vi "Write SAL_Events.vi"(8 "error in (no error)":errorcluster, 10 "SAL_Events.lvclass":refnum<class "SAL_Events.lvclass">, 11 "SAL_Listener in":refnum<class "SAL_Listener.lvclass">) -> (0 "error out":errorcluster, 3 "SAL_Listener out":refnum<class "SAL_Listener.lvclass">)   [LabVIEW 2016, in "SAL_Listener.lvclass"]
uses:
  SAL_Listener.lvclass
  SALEvents/SAL_Events.lvclass
  SAL_Listener.lvclass/SAL_Listener.ctl
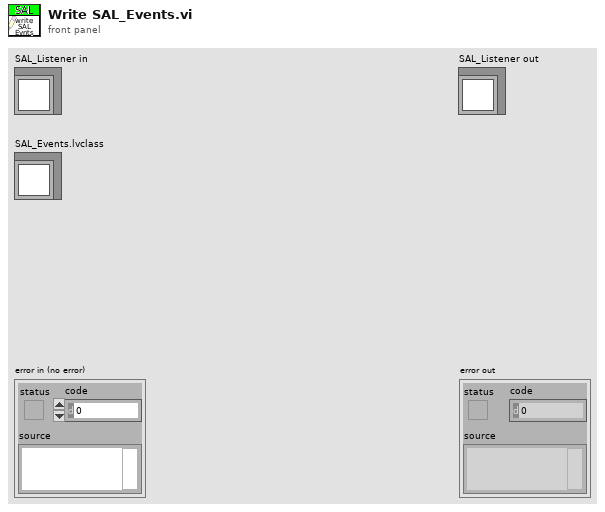
[diagram p1: front panel]
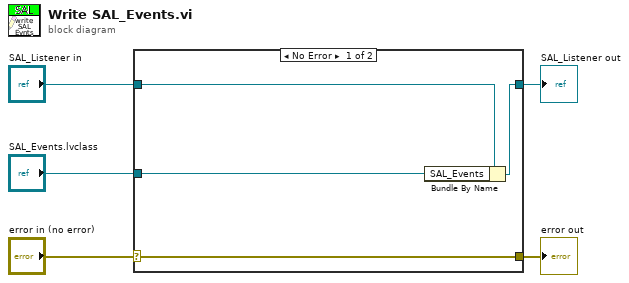
[diagram p0: block diagram]
diagram:
  n1 = case shown="No Error" "error in (no error)" {
    selector: "error in (no error)" -> [w9 w10]
    tunnel: [w9 w10] -> w4
    tunnel: [w7 w11] -> w2
    tunnel: "SAL_Listener in" -> [w8 w11]
    tunnel: "SAL_Events.lvclass" -> [w6 _]
    frame No Error {
      n2 = Bundle By Name(cluster=w8, "SAL_Events"=w6) -> (w7:refnum<class "SAL_Listener.lvclass">)
    }
    frame Error {
    }
  }
  "error out" <- w4
  "SAL_Listener out" <- w2
